vi "edittest Sequence STEPS.vi"(7 "Template Keys In (empty)":T1, 8 "error in (no error)":errorcluster, 10 "Sequence Id (\"\")":string, 11 "Connection Refnum":T2) -> (0 "error out":errorcluster, 3 "Connection Refnum":T2, 5 "Template Keys Out":T1)   [LabVIEW 2011]
uses:
  Summitek EXT/ODBC/SQL Controls/Connection Refnum.ctl
  ITK EXT/utils/keyedarr.llb/Keyed Array.ctl
  ITK EXT/utils/strutil.llb/Case Matching.ctl
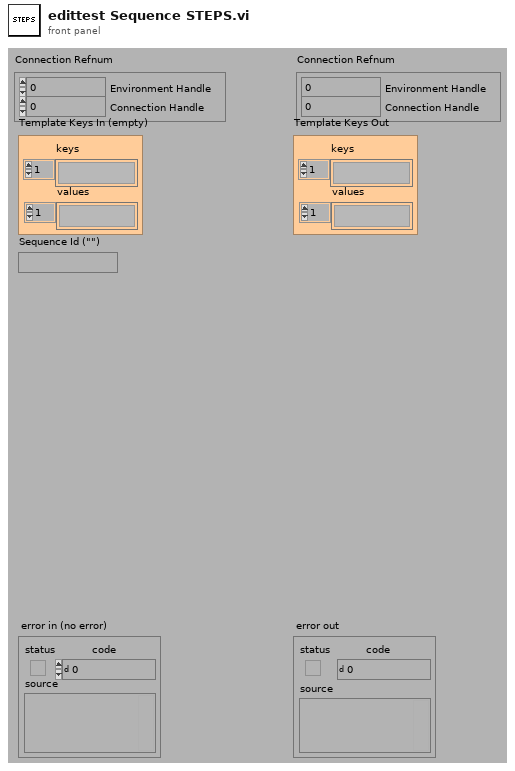
[diagram p1: front panel]
types:
  T1 = typedef "Keyed Array.ctl" = cluster{"keys":string[], "values":string[]}
  T2 = typedef "Connection Refnum.ctl" = cluster{"Environment Handle":i32, "Connection Handle":i32}
  T3 = typedef "Case Matching.ctl" = enum16{"a != A", "a == A", "system"}
  T4 = typedef "Test Record.ctl" = cluster{"ixTest":i32, "sxTestId":string, "sVersion":string, "sDriverTypes":string[], "sDescription":string, "iQuickMode":i32}
  T5 = typedef "Step Record.ctl" = cluster{"ixStep":i32, "sxSequenceId":string, "sxTestId":string, "iIndex":i32, "iRepeat":i32, "iQuickMode":i32, "sTag":string, "sDatasheetsCSV":string, "bConfiguration":string}
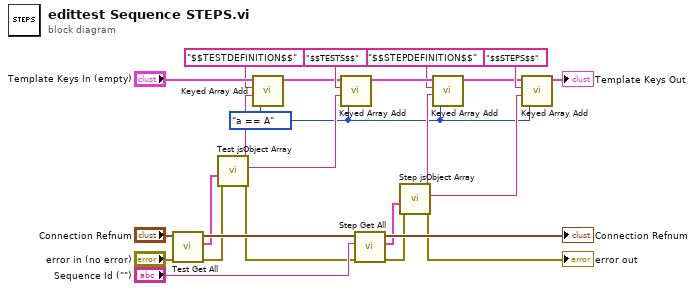
[diagram p0: block diagram]
diagram:
  w1 = Case_Matching."a == A" ("case matching (sensitive)")
  n1 = call "Test Get All.vi"("error in (no error)"="error in (no error)", "Connection Refnum"="Connection Refnum") -> ("error out"=w7:errorcluster, "Test Records"=w3:T4[], "Connection Refnum"=w22:T2)  [unwired: 2 in, 5 out]
  n2 = call "Test jsObject Array.vi"("error in (no error)"=w7, "TESTS (none)"=w3) -> ("error out"=w6:errorcluster, "Tests jsObject Array"=w5:string, "Test Definition"=w4:string)  [unwired: 2 in, 5 out]
  n3 = call "Keyed Array Add.vi"("case matching (sensitive)"=w1, "value"=w4, "key"="$$TESTDEFINITION$$", "array in"="Template Keys In (empty)") -> ("array out"=w9:T1)  [unwired: 3 out]
  n4 = call "Keyed Array Add.vi"("case matching (sensitive)"=w1, "value"=w5, "key"="$$TESTS$$", "array in"=w9) -> ("array out"=w15:T1)  [unwired: 3 out]
  n5 = call "Step Get All.vi"("error in (no error)"=w6, "sxSequenceId"="Sequence Id (\"\")", "Connection Refnum"=w22) -> ("error out"=w20:errorcluster, "Sequence Steps"=w2:T5[], "Connection Refnum"=→"Connection Refnum":T2)  [unwired: 1 in, 5 out]
  n6 = call "Step jsObject Array.vi"("error in (no error)"=w20, "STEPS (none)"=w2) -> ("error out"=→"error out":errorcluster, "Steps jsObject Array"=w11:string, "Step Definition"=w13:string)  [unwired: 3 in, 4 out]
  n7 = call "Keyed Array Add.vi"("case matching (sensitive)"=w1, "value"=w13, "key"="$$STEPDEFINITION$$", "array in"=w15) -> ("array out"=w14:T1)  [unwired: 3 out]
  n8 = call "Keyed Array Add.vi"("case matching (sensitive)"=w1, "value"=w11, "key"="$$STEPS$$", "array in"=w14) -> ("array out"=→"Template Keys Out":T1)  [unwired: 3 out]
